vi "PAG-CHECKCRC.vi"(10 "Array":u16[](array[numeric])=[100, 3, 0, 10, 0, 1] format="%02x") -> (2 "output array":u16[](array[numeric]) format="%02x")   [LabVIEW 2018]
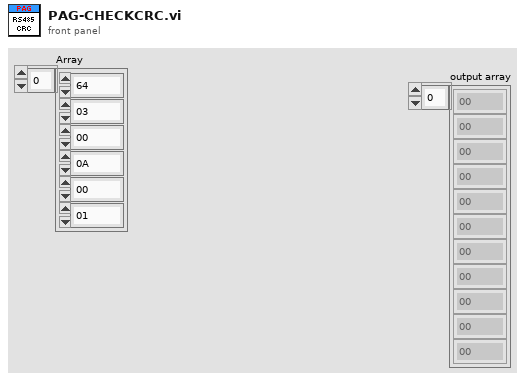
[diagram p1: front panel]
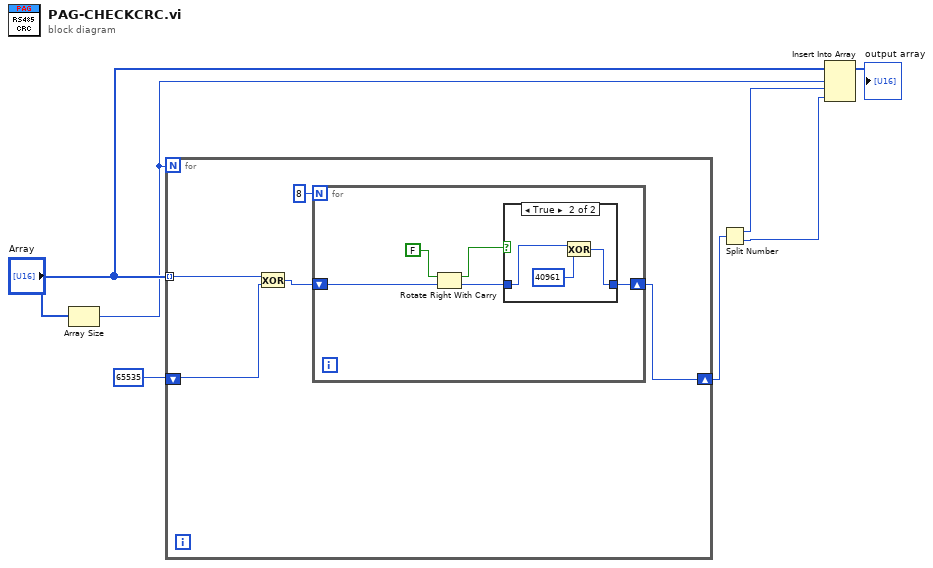
[diagram p0: block diagram]
diagram:
  n1 = Array Size(array="Array") -> (size(s)=w4:i32)
  n2 = for {
    N: w4 -> [_]
    tunnel: "Array" -> [w11] mode=indexing
    shift-right: [w8] -> w6
    shift-left: u16 65535 ("INITIAL") -> [w10]
    n3 = Exclusive Or(1:w10, 2:w11) -> (0:w9:u16)
    n4 = for {
      N: 8 -> [_]
      shift-right: [w13] -> w8
      shift-left: w9 -> [w16]
      n5 = Rotate Right With Carry(2:w16, 3:FALSE ("carry")) -> (0:w14:u16, 1:w15:bool)
      n6 = case shown="True" w15 {
        tunnel: w14 -> [w18 w21]
        tunnel: [w18 w19] -> w13
        frame False {
        }
        frame True {
          n7 = Exclusive Or(1:u16 40961 ("INITIAL"), 2:w21) -> (0:w19:u16)
        }
      }
    }
  }
  n8 = Split Number(x=w6) -> (hi(x)=w3:u8, lo(x)=w2:u8)
  n9 = Insert Into Array(array="Array", index=w4, new element #1=w3, new element #2=w2) -> (→"output array":u16[])
